vi "Close.vi"(8 "error in (no error)":errorcluster, 11 "OpenSSL Socket in":refnum<class "SSL Socket.lvclass">) -> (0 "error out":errorcluster)   [LabVIEW 2013, in "OpenSSL Socket.lvlib" / "SSL Socket.lvclass"]
doc: "Closes the socket connection.\nWebSockets 2.0.0.28\nSam Sharp - MediaMongrels Ltd\nCopyright (c) 2019, MediaMongrels Ltd"
uses:
  SSL Socket.lvclass
  SSL Socket.lvclass/SSL Socket.ctl
  SSL_Lib/BIO/BIO.lvclass
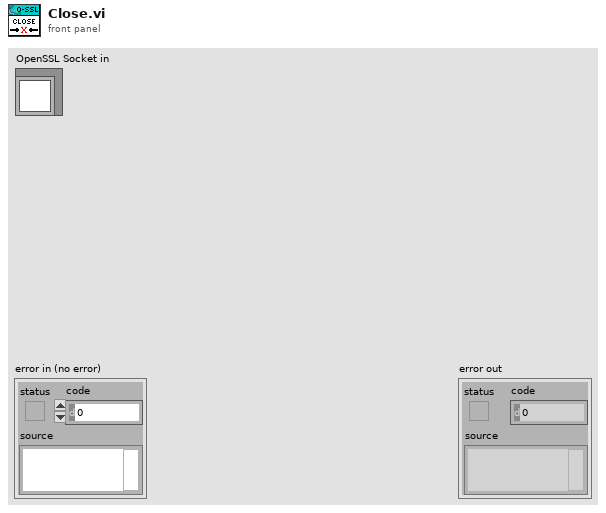
[diagram p1: front panel]
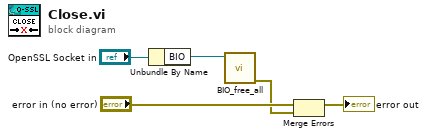
[diagram p0: block diagram]
diagram:
  n1 = Unbundle By Name("OpenSSL Socket in") -> ("BIO"=w2:refnum<class "BIO.lvclass">)
  n2 = call "BIO_free_all.vi"("BIO in"=w2) -> ("error out"=w1:errorcluster)  [unwired: 10 in]
  n3 = Merge Errors("error in (no error)", w1) -> (→"error out":errorcluster)
